vi "실습 5-4.vi"() -> ()   [LabVIEW 2014]
panel:
  in  "머신 이름(\"\":  로컬 참조 열기)":string
  in  "vi 경로":path
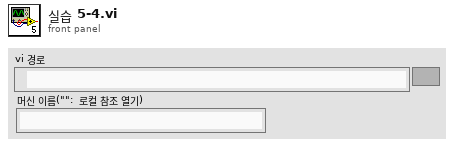
[diagram p1: front panel]
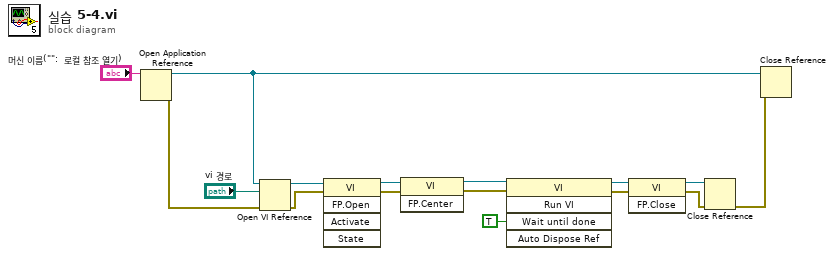
[diagram p0: block diagram]
diagram:
  n1 = Open Application Reference(11:"머신 이름(\"\":  로컬 참조 열기)") -> (0:w4:errorcluster, 3:w3:refnum<vi>)  [unwired: 3 in]
  n2 = Open VI Reference(application reference (local)=w3, vi path="vi 경로", error in (no error)=w4) -> (vi reference=w15:refnum<vi>, error out=w10:errorcluster)  [unwired: 3 in]
  n3 = invoke class="VI" method="FP.Open"(reference=w15, error in=w10) -> (reference out=w8:refnum<vi>, error out=w7:errorcluster)  [unwired: 3 in, 3 out]
  n4 = invoke class="VI" method="FP.Center"(reference=w8, error in=w7) -> (reference out=w6:refnum<vi>, error out=w5:errorcluster)  [unwired: 1 in, 1 out]
  n5 = invoke class="VI" method="Run VI"(reference=w6, error in=w5, "Wait until done"=TRUE ("완료될 때까지 기다림")) -> (reference out=w13:refnum<vi>, error out=w12:errorcluster)  [unwired: 2 in, 3 out]
  n6 = invoke class="VI" method="FP.Close"(reference=w13, error in=w12) -> (reference out=w11:refnum<vi>, error out=w9:errorcluster)  [unwired: 1 in, 1 out]
  n7 = Close Reference(reference=w11, error in (no error)=w9) -> (error out=w1:errorcluster)
  n8 = Close Reference(reference=w3, error in (no error)=w1) -> ()  [unwired: 1 out]
